vi "Clear Register .vi"(8 "error in (no error)":errorcluster, 11 "VISA resource name":refnum<visa-resource-name>) -> (0 "error out":errorcluster, 3 "VISA resource name out":refnum<visa-resource-name>)   [LabVIEW 2021, in "Agilent 532XX Series.lvlib"]
doc: "Clears all bits in the Questionable Data enable register and the Standard Operation enable register."
uses:
  <instrlib>/Agilent 532XX Series/Agilent 532XX Series.lvlib
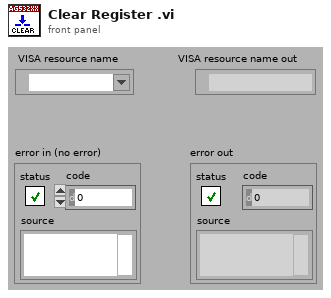
[diagram p1: front panel]
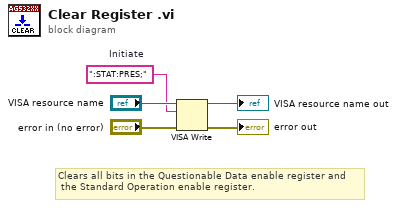
[diagram p0: block diagram]
diagram:
  w3 = ":STAT:PRES;"  # Initiate
  # "Clears all bits in the Questionable Data enable register and\n the Standard Operation enable register."
  n1 = VISA Write(VISA resource name="VISA resource name", write buffer=w3, error in (no error)="error in (no error)") -> (VISA resource name out=→"VISA resource name out":refnum<visa-resource-name>, error out=→"error out":errorcluster)  [unwired: 1 out]
